vi "Periodic Tasks.vi"(8 "error in":errorcluster) -> ()   [LabVIEW 2016]
doc: "This VI runs in parallel to other robot code. It can contain as many user-defined periodic loops as you need. These can carry out PID or other sorts of timed response."
uses:
  <vilib>/Rock Robotics/WPI/Utilities/WPI_GetSetVariantRefNum.vi
  Robot Global Data.vi
  Support Code/Team900-VIs/navX Library v2/navX Library v2.lvlib
panel:
  in  "Zero Yaw":bool=TRUE
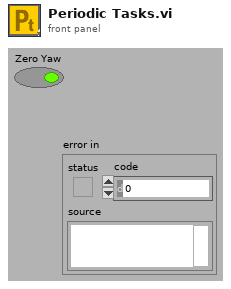
[diagram p1: front panel]
types:
  T1 = typedef "WPI_JoystickDevRef.ctl" = cluster{"Device":T2}
  T2 = typedef "WPI_JoystickDeviceEnum.ctl" = enum16{"USB 0", "USB 1", "USB 2", "USB 3", "USB 4", "USB 5"}
  T3 = typedef "navX Library v2.lvlib/Z900_navX_DeviceTypeDef.ctl" = cluster{"Interface":cluster{"Protocol":T4, "Update Rate (4Hz-60Hz)":u8, "navX Open TypeDef":variant}, "Notify Packet":refnum<notifier>, "Loop VI Refnum":refnum<vi>, "Ready to Close Occurrence Refnum":refnum<k4>}
  T4 = typedef "navX Library v2.lvlib/Z900_navX_ProtocolTypeDef.ctl" = enum16{"SERIAL", "I2C", "SPI"}
  T5 = cluster{"Yaw":dbl, "Roll":dbl, "Pitch":dbl, "Heading":dbl, "Fused Heading":dbl}
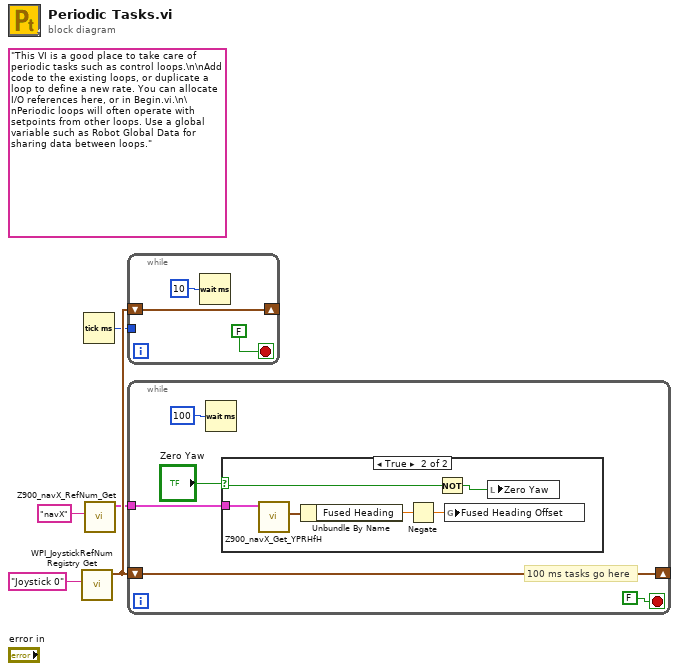
[diagram p0: block diagram]
diagram:
  (unwired) "This VI is a good place to take care of periodic tasks such as control loops.\n\nAdd code to the existing loops, or duplicate a loop to define a new rate. You can allocate I/O references here, or in Begin.vi.\n\nPeriodic loops will often operate with setpoints from other loops. Use a global variable such as Robot Global Data for sharing data between loops."
  n1 = call <vilib>:"WPI_JoystickRefNum Registry Get.vi"("refnum name"="Joystick 0") -> ("JoystickDevRef"=w4:T1)  [unwired: 1 in, 9 out]
  n2 = Tick Count (ms)() -> (millisecond timer value=w3:u32)
  n3 = call "Z900_navX_RefNum_Get.vi"("refnum name"="navX") -> ("navX Device"=w1:T3)  [unwired: 9 in, 1 out]
  n4 = while {
    shift-right: [w7] -> _
    shift-left: w4 -> [w7]
    tunnel: w3 -> [_]
    stop <- FALSE stop-if-true
    n5 = Wait (ms)(milliseconds to wait=u32 10) -> ()  [unwired: 1 out]
  }
  n6 = while {
    shift-right: [w11] -> _
    shift-left: w4 -> [w11]
    tunnel: w1 -> [w10]
    stop <- FALSE stop-if-true
    # "100 ms tasks go here"
    n7 = Wait (ms)(milliseconds to wait=u32 100) -> ()  [unwired: 1 out]
    n8 = case shown="True" "Zero Yaw" {
      selector: "Zero Yaw" -> [_ w15]
      tunnel: w10 -> [_ w19]
      frame False {
      }
      frame True {
        n9 = call "Z900_navX_Get_YPRHfH.vi"("navX Device"=w19) -> ("YRPHfH"=w18:T5)  [unwired: 7 in, 3 out]
        n10 = Unbundle By Name(w18) -> ("Fused Heading"=w17:dbl)
        n11 = Negate(x=w17) -> (-x=w16:dbl)
        n12 = Not(x=w15) -> (.not. x?=w14:bool)
        n13 = global write "Robot Global Data.vi" "Fused Heading Offset"(w16) -> ()
        n14 = local write "Zero Yaw"(w14) -> ()
      }
    }
  }
